vi "comicvine.to.local_publisher.vi"(8 "error in (no error)":errorcluster, 11 "cv publisher":T1) -> (0 "error out":errorcluster, 3 "local publisher":T4)   [LabVIEW 2024]
uses:
  definitions/local_publisher.ctl
  definitions/comicvine_publisher.ctl
  definitions/comicvine_publisher.results.ctl
  definitions/comicvine_volume.issue.ctl
  <userlib>/_OpenG.lib/string/string.llb/openg_string.lvlib
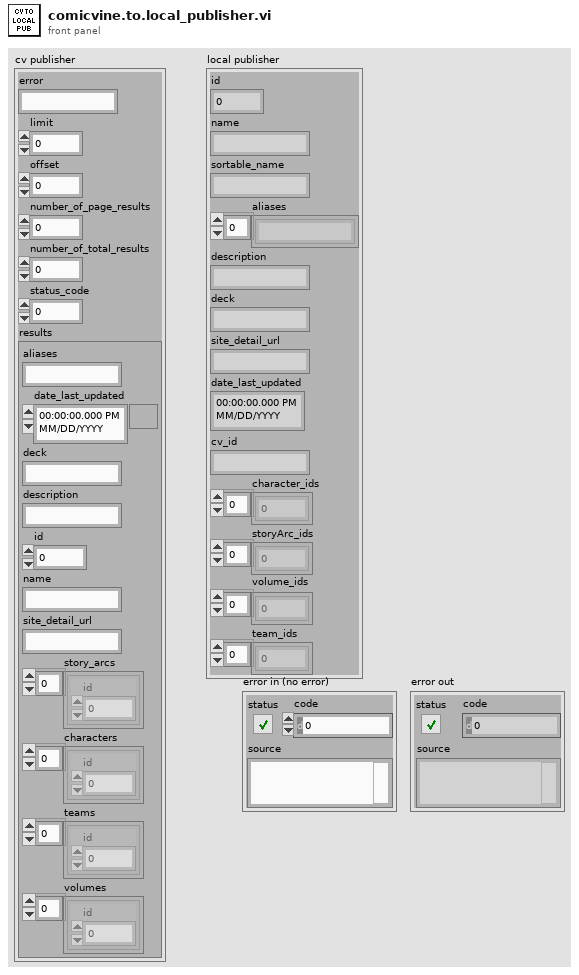
[diagram p1: front panel]
types:
  T1 = typedef "comicvine_publisher.ctl" = cluster{"error":string, "limit":i32, "offset":i32, "number_of_page_results":i32, "number_of_total_results":i32, "status_code":i32, "results":T2}
  T2 = typedef "comicvine_publisher.results.ctl" = cluster{"aliases":string, "date_last_updated":timestamp, "deck":string, "description":string, "id":i32, "name":string, "site_detail_url":string, "story_arcs":T3[], "characters":T3[], "teams":T3[], "volumes":T3[]}
  T3 = typedef "comicvine_volume.issue.ctl" = cluster{"id":i32}
  T4 = typedef "local_publisher.ctl" = cluster{"id":i32, "name":string, "sortable_name":string, "aliases":string[], "description":string, "deck":string, "site_detail_url":string, "date_last_updated":timestamp, "cv_id":string, "character_ids":i32[], "storyArc_ids":i32[], "volume_ids":i32[], "team_ids":i32[]}
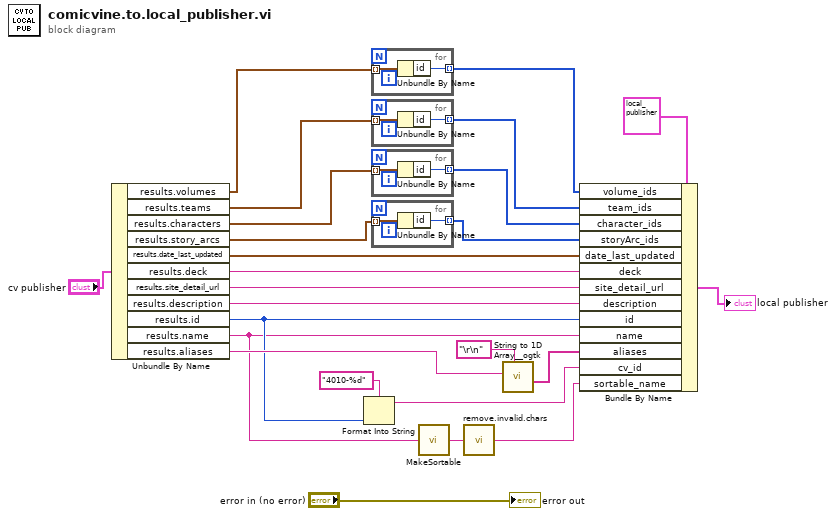
[diagram p0: block diagram]
diagram:
  n1 = Unbundle By Name("cv publisher") -> ("results.volumes"=w1:T3[], "results.teams"=w2:T3[], "results.characters"=w16:T3[], "results.story_arcs"=w6:T3[], "results.date_last_updated"=w7:timestamp, "results.deck"=w9:string, "results.site_detail_url"=w17:string, "results.description"=w18:string, "results.id"=w13:i32, "results.name"=w10:string, "results.aliases"=w21:string)
  n2 = Format Into String(format string="4010-%d", w13) -> (resulting string=w12:string)  [unwired: 2 in, 1 out]
  n3 = for {
    tunnel: w1 -> [w27] mode=indexing
    tunnel: [w26] -> w3 mode=indexing
    n4 = Unbundle By Name(w27) -> ("id"=w26:i32)
  }
  n5 = for {
    tunnel: w2 -> [w29] mode=indexing
    tunnel: [w28] -> w4 mode=indexing
    n6 = Unbundle By Name(w29) -> ("id"=w28:i32)
  }
  n7 = for {
    tunnel: w16 -> [w31] mode=indexing
    tunnel: [w30] -> w15 mode=indexing
    n8 = Unbundle By Name(w31) -> ("id"=w30:i32)
  }
  n9 = for {
    tunnel: w6 -> [w33] mode=indexing
    tunnel: [w32] -> w5 mode=indexing
    n10 = Unbundle By Name(w33) -> ("id"=w32:i32)
  }
  n11 = call "MakeSortable.vi"("string in"=w10) -> ("string out"=w22:string)
  n12 = call "remove.invalid.chars.vi"("string in"=w22) -> ("string out"=w8:string)
  n13 = call <userlib>:"String to 1D Array__ogtk.vi"("delimiter (Tab)"="\r\n", "string"=w21) -> ("Array of Strings"=w19:string[])  [unwired: 9 in]
  n14 = Bundle By Name(cluster=T4 {"id"=0, "name"="", "sortable_name"="", "aliases"=[], "description"="", "deck"="", "site_detail_url"="", "date_last_updated"=timestamp(0 s since 1904-01-01), "cv_id"="", "character_ids"=[], "storyArc_ids"=[], "volume_ids"=[], "team_ids"=[]} ("local publisher"), "volume_ids"=w3, "team_ids"=w4, "character_ids"=w15, "storyArc_ids"=w5, "date_last_updated"=w7, "deck"=w9, "site_detail_url"=w17, "description"=w18, "id"=w13, "name"=w10, "aliases"=w19, "cv_id"=w12, "sortable_name"=w8) -> (→"local publisher":T4)
  "error out" <- "error in (no error)"
